vi "ELVIS III v1.0 Configure DO ENA.vi"(5 "Apply Bitmask?":bool=TRUE, 7 "Connector List":T1, 8 "error in (no error)":errorcluster, 10 "Bitmask Array":bool[](array[boolean]), 11 "myRIO FPGA Ref In":T2) -> (0 "error out":errorcluster)   [LabVIEW 2021]
uses:
  <vilib>/myRIO/Common/Instrument Driver Framework/Utilities/typedefs/Generic FPGA Reference.ctl
  <vilib>/myRIO/Common/Instrument Driver Framework/ELVIS III v1.0/Resource Manager/typedefs/ELVIS III v1.0 Connector List.ctl
  <vilib>/myRIO/Common/Instrument Driver Framework/ELVIS III v1.0/DO Block/typedefs/ELVIS III DO Block FPGA Reference.ctl
  <vilib>/Utility/error.llb/Error Cluster From Error Code.vi
  <vilib>/rvi/errors/niLvFpgaAdjustHostInterfaceError.vi
  <vilib>/rvi/interface/nirviReadWriteControl/nirviReadWriteControl.xnode
  NiFpgaLv.dll
  <vilib>/rvi/interface/Simulation/niFpgaSimulationCallBeginRW.vi
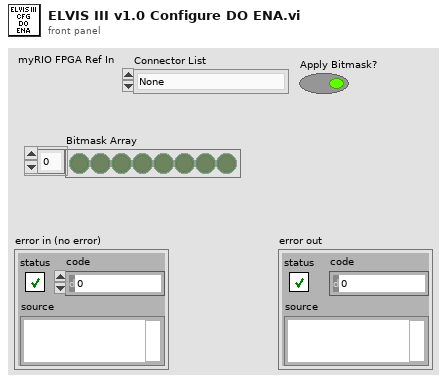
[diagram p1: front panel]
types:
  T1 = typedef "ELVIS III v1.0 Connector List.ctl" = enum32{"None", "ConnectorA", "ConnectorB"}
  T2 = typedef "Generic FPGA Reference.ctl" = refnum<k20>
  T3 = typedef "ELVIS III DO Block FPGA Reference.ctl" = refnum<k20>
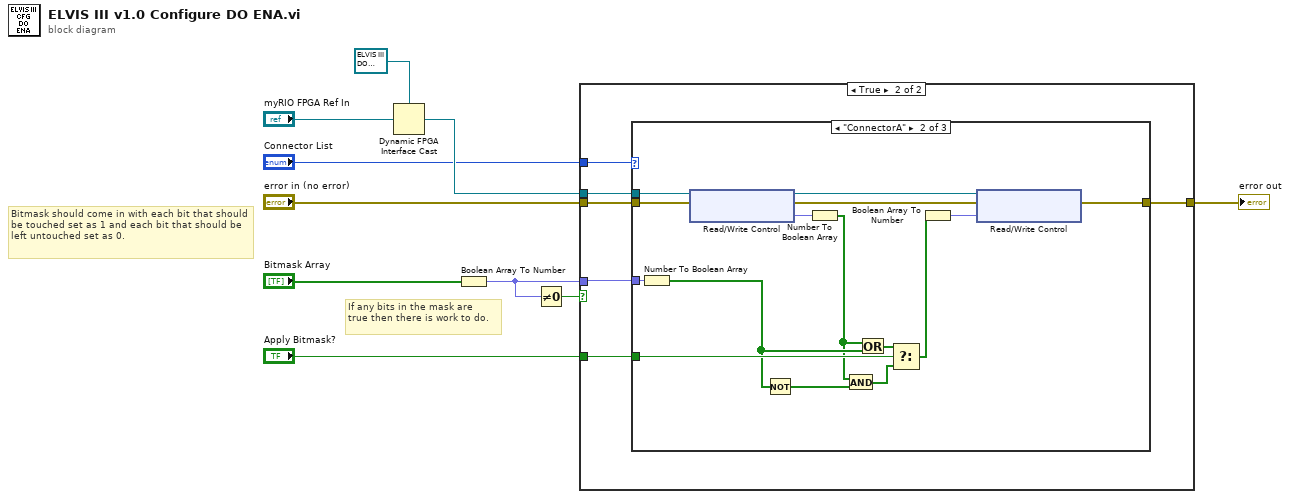
[diagram p0: block diagram]
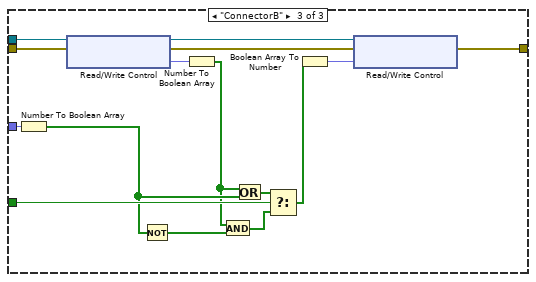
[diagram p4: hidden frame]
diagram:
  # "If any bits in the mask are\ntrue then there is work to do."
  # "Bitmask should come in with each bit that should be touched set as 1 and each bit that should be left untouched set as 0."
  n1 = Dynamic FPGA Interface Cast(Session In=T3 refnum ("FPGA Interface"), Type="myRIO FPGA Ref In") -> (Session Out=w7:T3)
  n2 = Boolean Array To Number(Boolean array="Bitmask Array") -> (number=w3:fxp<+,20,20>)
  n3 = Not Equal To 0?(x=w3) -> (x != 0?=w2:bool)
  n4 = case shown="True" w2 {
    tunnel: w7 -> [_ w17]
    tunnel: "error in (no error)" -> [w11 w16]
    tunnel: [w11 w15] -> w9
    tunnel: w3 -> [_ w14]
    tunnel: "Apply Bitmask?" -> [_ w13]
    tunnel: "Connector List" -> [_ w12]
    frame False {
      # "There are no bits to change for this connector."
    }
    frame True {
      n5 = case shown="\"ConnectorA\"" w12 {
        tunnel: w17 -> [_ w32 w47]
        tunnel: w16 -> [w18 w33 w48]
        tunnel: [w18 w19 w34] -> w15
        tunnel: w14 -> [_ w30 w45]
        tunnel: w13 -> [_ w31 w46]
        frame "None", Default {
          # "Do Nothing"
        }
        frame "ConnectorA" {
          n6 = Number To Boolean Array(number=w30) -> (Boolean array=w29:bool[])
          n7 = xnode "Read/Write Control"("FPGA VI Reference In"=w32, "error in"=w33) -> ("FPGA VI Reference Out"=w26:T3, "error out"=w27:errorcluster, "DO.A.DMA_ENA"=w28:fxp<+,20,20>)
          n8 = Not(x=w29) -> (.not. x?=w24:bool[])
          n9 = Number To Boolean Array(number=w28) -> (Boolean array=w22:bool[])
          n10 = And(x=w22, y=w24) -> (x .and. y?=w23:bool[])
          n11 = Or(x=w22, y=w29) -> (x .or. y?=w25:bool[])
          n12 = Select(t=w25, s=w31, f=w23) -> (s? t:f=w21:bool[])
          n13 = Boolean Array To Number(Boolean array=w21) -> (number=w20:fxp<+,20,20>)
          n14 = xnode "Read/Write Control"("FPGA VI Reference In"=w26, "error in"=w27, "DO.A.DMA_ENA"=w20) -> ("error out"=w19:errorcluster)  [unwired: 1 out]
        }
        frame "ConnectorB" {
          n15 = Number To Boolean Array(number=w45) -> (Boolean array=w44:bool[])
          n16 = xnode "Read/Write Control"("FPGA VI Reference In"=w47, "error in"=w48) -> ("FPGA VI Reference Out"=w41:T3, "error out"=w42:errorcluster, "DO.B.DMA_ENA"=w43:fxp<+,20,20>)
          n17 = Not(x=w44) -> (.not. x?=w39:bool[])
          n18 = Number To Boolean Array(number=w43) -> (Boolean array=w37:bool[])
          n19 = And(x=w37, y=w39) -> (x .and. y?=w38:bool[])
          n20 = Or(x=w37, y=w44) -> (x .or. y?=w40:bool[])
          n21 = Select(t=w40, s=w46, f=w38) -> (s? t:f=w36:bool[])
          n22 = Boolean Array To Number(Boolean array=w36) -> (number=w35:fxp<+,20,20>)
          n23 = xnode "Read/Write Control"("FPGA VI Reference In"=w41, "error in"=w42, "DO.B.DMA_ENA"=w35) -> ("error out"=w34:errorcluster)  [unwired: 1 out]
        }
      }
    }
  }
  "error out" <- w9
